vi "IMAQdx Write Memory.vi"(8 "error in":errorcluster, 9 "Value":string, 10 "Offset":u32=4042262528 format="%.0x", 11 "Session In":T1) -> (0 "error out":errorcluster, 3 "Session Out":T1)   [LabVIEW 2020, in "NI_Vision_Acquisition_Software.lvlib"]
doc: "Accesses registers on the camera and writes a string to the camera."
uses:
  NI_Vision_Acquisition_Software.lvlib
  IMAQdx.ctl
  niimaqdx.dll
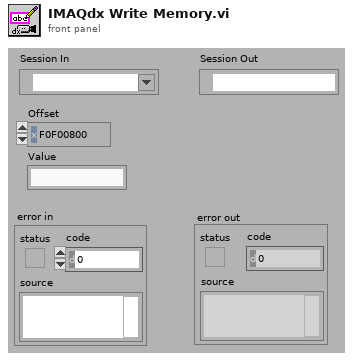
[diagram p1: front panel]
types:
  T1 = typedef "IMAQdx.ctl" = refnum<k21>
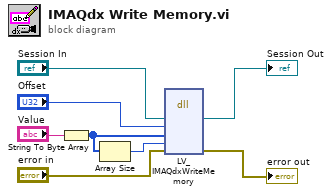
[diagram p0: block diagram]
diagram:
  n1 = String To Byte Array(string="Value") -> (unsigned byte array=w2:u8[])
  n2 = Array Size(array=w2) -> (size(s)=w1:i32)
  n3 = dll-call lib="niimaqdx.dll" fn="LV_IMAQdxWriteMemory"("Session In"="Session In", "offset"="Offset", "array"=w2, "count"=w1, "error in"="error in") -> ("Session In"=→"Session Out":T1, "error in"=→"error out":errorcluster)  [unwired: 7 in, 2 out]
